vi "ClimberLogic.vi"   [LabVIEW 2020]
uses:
  Robot Global Data.vi
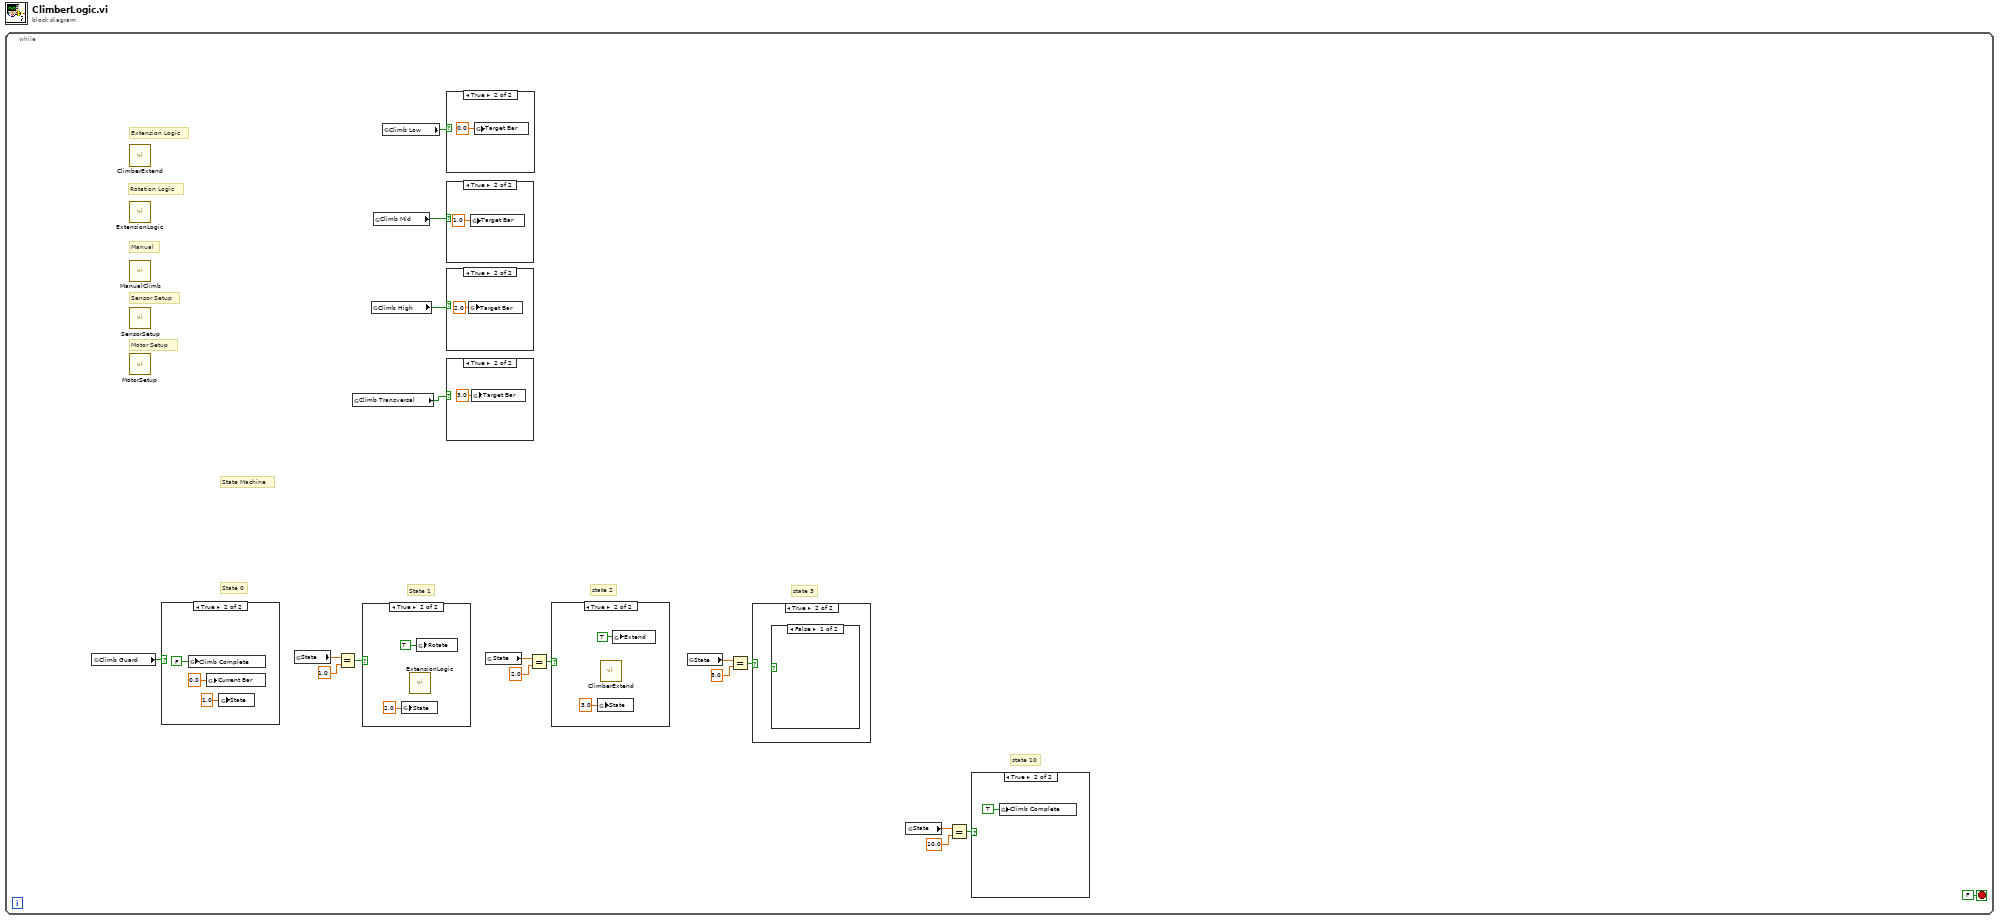
[diagram p0: block diagram]
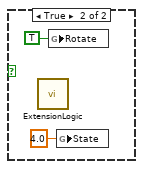
[diagram p4: hidden frame]
diagram:
  n1 = while {
    stop <- FALSE stop-if-true
    # "state 10"
    # "state 3"
    # "state 2"
    # "State 1"
    # "State 0"
    # "State Machine"
    # "Motor Setup"
    # "Extension Logic"
    # "Rotation Logic"
    # "Manual"
    # "Sensor Setup"
    n2 = global read "Robot Global Data.vi" "Climb Guard"() -> (w13:bool)
    n3 = call "ClimberExtend.vi"() -> ()  [unwired: 12 in]
    n4 = call "ExtensionLogic.vi"() -> ()  [unwired: 12 in]
    n5 = call "MotorSetup.vi"() -> ()  [unwired: 12 in]
    n6 = call "ManualClimb.vi"() -> ()  [unwired: 12 in]
    n7 = call "SensorSetup.vi"() -> ()  [unwired: 12 in]
    n8 = case shown="True" w13 {
      frame False {
      }
      frame True {
        n9 = global write "Robot Global Data.vi" "Climb Complete"(FALSE ("Climb Complete")) -> ()
        n10 = global write "Robot Global Data.vi" "Current Bar"(0.0 ("Current Bar")) -> ()
        n11 = global write "Robot Global Data.vi" "State"(1.0 ("State")) -> ()
      }
    }
    n12 = global read "Robot Global Data.vi" "State"() -> (w12:dbl)
    n13 = Equal?(x=w12, y=1.0) -> (x = y?=w10:bool)
    n14 = global read "Robot Global Data.vi" "Climb Transversal"() -> (w14:bool)
    n15 = case shown="True" w10 {
      frame False {
      }
      frame True {
        n16 = global write "Robot Global Data.vi" "State"(2.0 ("State")) -> ()
        n17 = call "ExtensionLogic.vi"() -> ()  [unwired: 12 in]
        n18 = global write "Robot Global Data.vi" "Rotate"(TRUE ("Rotate")) -> ()
      }
    }
    n19 = global read "Robot Global Data.vi" "Climb High"() -> (w15:bool)
    n20 = global read "Robot Global Data.vi" "Climb Mid"() -> (w16:bool)
    n21 = global read "Robot Global Data.vi" "Climb Low"() -> (w17:bool)
    n22 = case shown="True" w16 {
      frame False {
      }
      frame True {
        n23 = global write "Robot Global Data.vi" "Target Bar"(1.0 ("Target Bar")) -> ()
      }
    }
    n24 = case shown="True" w15 {
      frame False {
      }
      frame True {
        n25 = global write "Robot Global Data.vi" "Target Bar"(2.0 ("Target Bar")) -> ()
      }
    }
    n26 = case shown="True" w14 {
      frame False {
      }
      frame True {
        n27 = global write "Robot Global Data.vi" "Target Bar"(3.0 ("Target Bar")) -> ()
      }
    }
    n28 = case shown="True" w17 {
      frame False {
      }
      frame True {
        n29 = global write "Robot Global Data.vi" "Target Bar"(0.0 ("Target Bar")) -> ()
      }
    }
    n30 = global read "Robot Global Data.vi" "State"() -> (w9:dbl)
    n31 = Equal?(x=w9, y=2.0) -> (x = y?=w7:bool)
    n32 = case shown="True" w7 {
      frame False {
      }
      frame True {
        n33 = global write "Robot Global Data.vi" "State"(3.0 ("State")) -> ()
        n34 = call "ClimberExtend.vi"() -> ()  [unwired: 12 in]
        n35 = global write "Robot Global Data.vi" "Extend"(TRUE ("Rotate")) -> ()
      }
    }
    n36 = global read "Robot Global Data.vi" "State"() -> (w6:dbl)
    n37 = Equal?(x=w6, y=3.0) -> (x = y?=w4:bool)
    n38 = case shown="True" w4 {
      frame False {
      }
      frame True {
        n39 = case shown="False" {
          selector: _ -> [_ _]
          frame False {
          }
          frame True {
            n40 = call "ExtensionLogic.vi"() -> ()  [unwired: 12 in]
            n41 = global write "Robot Global Data.vi" "Rotate"(TRUE ("Rotate")) -> ()
            n42 = global write "Robot Global Data.vi" "State"(4.0 ("State")) -> ()
          }
        }
      }
    }
    n43 = global read "Robot Global Data.vi" "State"() -> (w3:dbl)
    n44 = Equal?(x=w3, y=10.0) -> (x = y?=w1:bool)
    n45 = case shown="True" w1 {
      frame False {
      }
      frame True {
        n46 = global write "Robot Global Data.vi" "Climb Complete"(TRUE ("Climb Complete")) -> ()
      }
    }
  }
